vi "Apply Waveform Attributes.vi"(0 "RFSG Session In":refnum<k15>, 5 "Waveform":T1 {"Runtime Scaling" format="%#_6p"; "Sample Rate" format="%#_6p"; "Burst Length (s)" format="%#_6p"; "PAPR (dB)" format="%.2f"; "Signal Bandwidth (Hz)" format="%#_6p"}, 11 "error in (no error)":errorcluster) -> (4 "RFSG Session Out":refnum<k15>, 15 "error out":errorcluster)   [LabVIEW 2019, in "SG.lvlib"]
doc: "Calls <b>niRFSGPlayback Set Script To Generate (1 RFSG)</b>, which will download the script contained in waveform and apply all associated parameters."
uses:
  SG.lvlib
  Common/Waveform.ctl
  <instrlib>/niRFSGPlayback/niRFSGPlayback Set Script to Generate (1 RFSG).vi
  Common/Common.lvlib
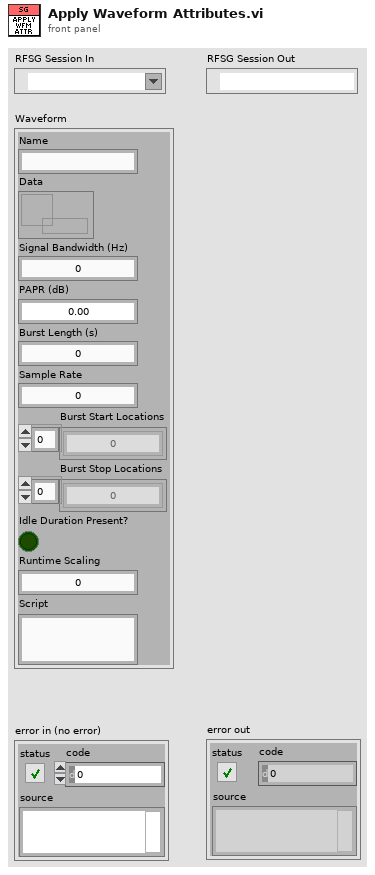
[diagram p1: front panel]
types:
  T1 = typedef "Common.lvlib/Waveform.ctl" = cluster{"Name":string, "Data":refnum<data-value>, "Signal Bandwidth (Hz)":dbl, "PAPR (dB)":dbl, "Burst Length (s)":dbl, "Sample Rate":dbl, "Burst Start Locations":i32[], "Burst Stop Locations":i32[], "Idle Duration Present?":bool, "Runtime Scaling":dbl, "Script":string}
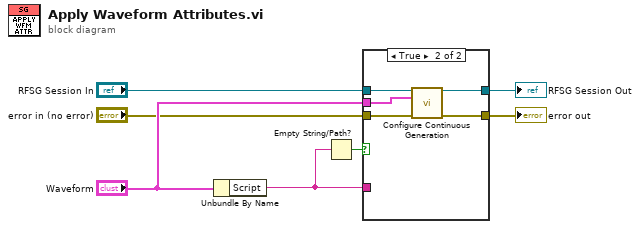
[diagram p0: block diagram]
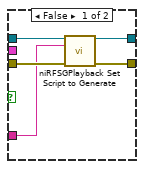
[diagram p2: hidden frame]
diagram:
  n1 = Unbundle By Name("Waveform") -> ("Script"=w1:string)
  n2 = Empty String/Path?(string/path=w1) -> (empty?=w6:bool)
  n3 = case shown="True" w6 {
    tunnel: "RFSG Session In" -> [w12 w17]
    tunnel: "Waveform" -> [_ w16]
    tunnel: "error in (no error)" -> [w11 w15]
    tunnel: [w8 w14] -> w3
    tunnel: [w9 w13] -> w2
    tunnel: w1 -> [w10 _]
    frame False {
      n4 = call-poly <instrlib>:"niRFSGPlayback Set Script to Generate.vi"("instrument handle in"=w12, "script text"=w10, "error in"=w11) -> ("instrument handle out"=w9:refnum<k15>, "error out"=w8:errorcluster)  [unwired: 11 in]
    }
    frame True {
      n5 = call "Configure Continuous Generation.vi"("RFSG handle"=w17, "Waveform in"=w16, "error in"=w15) -> ("RFSG handle out"=w13:refnum<k15>, "error out"=w14:errorcluster)  [unwired: 10 in, 1 out]
    }
  }
  "error out" <- w3
  "RFSG Session Out" <- w2
